vi "PulseDetectAndSwitch10.vi"(9 "Laser bits in":bool[](array[boolean])=[FALSE, FALSE, FALSE, FALSE, FALSE, FALSE, FALSE, FALSE, FALSE, FALSE], 10 "Last region":bool=TRUE, 11 "Last laser bit in":bool) -> (1 "Region array out":bool[](array[boolean]), 2 "New last region out":bool, 3 "New last laser bit out":bool)   [LabVIEW 2012]
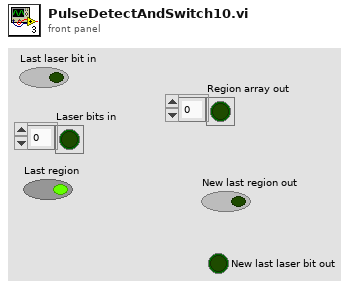
[diagram p1: front panel]
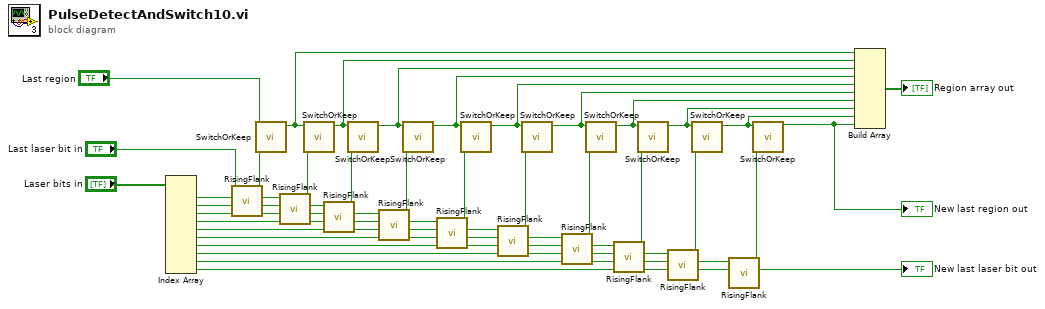
[diagram p0: block diagram]
diagram:
  n1 = Index Array(array="Laser bits in") -> (element #1=w32:bool, element #2=w31:bool, element #3=w30:bool, element #4=w29:bool, element #5=w28:bool, element #6=w27:bool, element #7=w26:bool, element #8=w25:bool, element #9=w24:bool, element #10=w1:bool)  [unwired: 10 in]
  "New last laser bit out" <- w1
  n2 = call "RisingFlank.vi"("2nd sample"=w32, "1st sample"="Last laser bit in") -> ("Rising flank?"=w22:bool)  [unwired: 7 in]
  n3 = call "SwitchOrKeep.vi"("Rising flank? in"=w22, "Last state in"="Last region") -> ("New state out"=w12:bool)  [unwired: 9 in]
  n4 = call "RisingFlank.vi"("2nd sample"=w31, "1st sample"=w32) -> ("Rising flank?"=w21:bool)  [unwired: 7 in]
  n5 = call "SwitchOrKeep.vi"("Rising flank? in"=w21, "Last state in"=w12) -> ("New state out"=w11:bool)  [unwired: 9 in]
  n6 = call "RisingFlank.vi"("2nd sample"=w30, "1st sample"=w31) -> ("Rising flank?"=w20:bool)  [unwired: 7 in]
  n7 = call "SwitchOrKeep.vi"("Rising flank? in"=w20, "Last state in"=w11) -> ("New state out"=w10:bool)  [unwired: 9 in]
  n8 = call "RisingFlank.vi"("2nd sample"=w29, "1st sample"=w30) -> ("Rising flank?"=w19:bool)  [unwired: 7 in]
  n9 = call "SwitchOrKeep.vi"("Rising flank? in"=w19, "Last state in"=w10) -> ("New state out"=w9:bool)  [unwired: 9 in]
  n10 = call "RisingFlank.vi"("2nd sample"=w28, "1st sample"=w29) -> ("Rising flank?"=w18:bool)  [unwired: 7 in]
  n11 = call "SwitchOrKeep.vi"("Rising flank? in"=w18, "Last state in"=w9) -> ("New state out"=w8:bool)  [unwired: 9 in]
  n12 = call "RisingFlank.vi"("2nd sample"=w27, "1st sample"=w28) -> ("Rising flank?"=w17:bool)  [unwired: 7 in]
  n13 = call "SwitchOrKeep.vi"("Rising flank? in"=w17, "Last state in"=w8) -> ("New state out"=w7:bool)  [unwired: 9 in]
  n14 = call "RisingFlank.vi"("2nd sample"=w26, "1st sample"=w27) -> ("Rising flank?"=w16:bool)  [unwired: 7 in]
  n15 = call "SwitchOrKeep.vi"("Rising flank? in"=w16, "Last state in"=w7) -> ("New state out"=w6:bool)  [unwired: 9 in]
  n16 = call "RisingFlank.vi"("2nd sample"=w25, "1st sample"=w26) -> ("Rising flank?"=w15:bool)  [unwired: 7 in]
  n17 = call "SwitchOrKeep.vi"("Rising flank? in"=w15, "Last state in"=w6) -> ("New state out"=w5:bool)  [unwired: 9 in]
  n18 = call "RisingFlank.vi"("2nd sample"=w24, "1st sample"=w25) -> ("Rising flank?"=w14:bool)  [unwired: 7 in]
  n19 = call "SwitchOrKeep.vi"("Rising flank? in"=w14, "Last state in"=w5) -> ("New state out"=w4:bool)  [unwired: 9 in]
  n20 = call "RisingFlank.vi"("2nd sample"=w1, "1st sample"=w24) -> ("Rising flank?"=w13:bool)  [unwired: 7 in]
  n21 = call "SwitchOrKeep.vi"("Rising flank? in"=w13, "Last state in"=w4) -> ("New state out"=w3:bool)  [unwired: 9 in]
  "New last region out" <- w3
  n22 = Build Array(w12, w11, w10, w9, w8, w7, w6, w5, w4, w3) -> (→"Region array out":bool[])
